vi "TSCAN_SetSignalValue_CANFD.vi"(6 "SigValue":dbl, 7 "TLIBCANFD":T1, 8 "错误输入（无错误）":errorcluster, 9 "Signal":string, 10 "CANFD Message":string, 11 "路径输入":path) -> (0 "错误输出":errorcluster, 1 "CANFDObJ":T1, 2 "return":i32, 3 "路径输出":path)   [LabVIEW 2014]
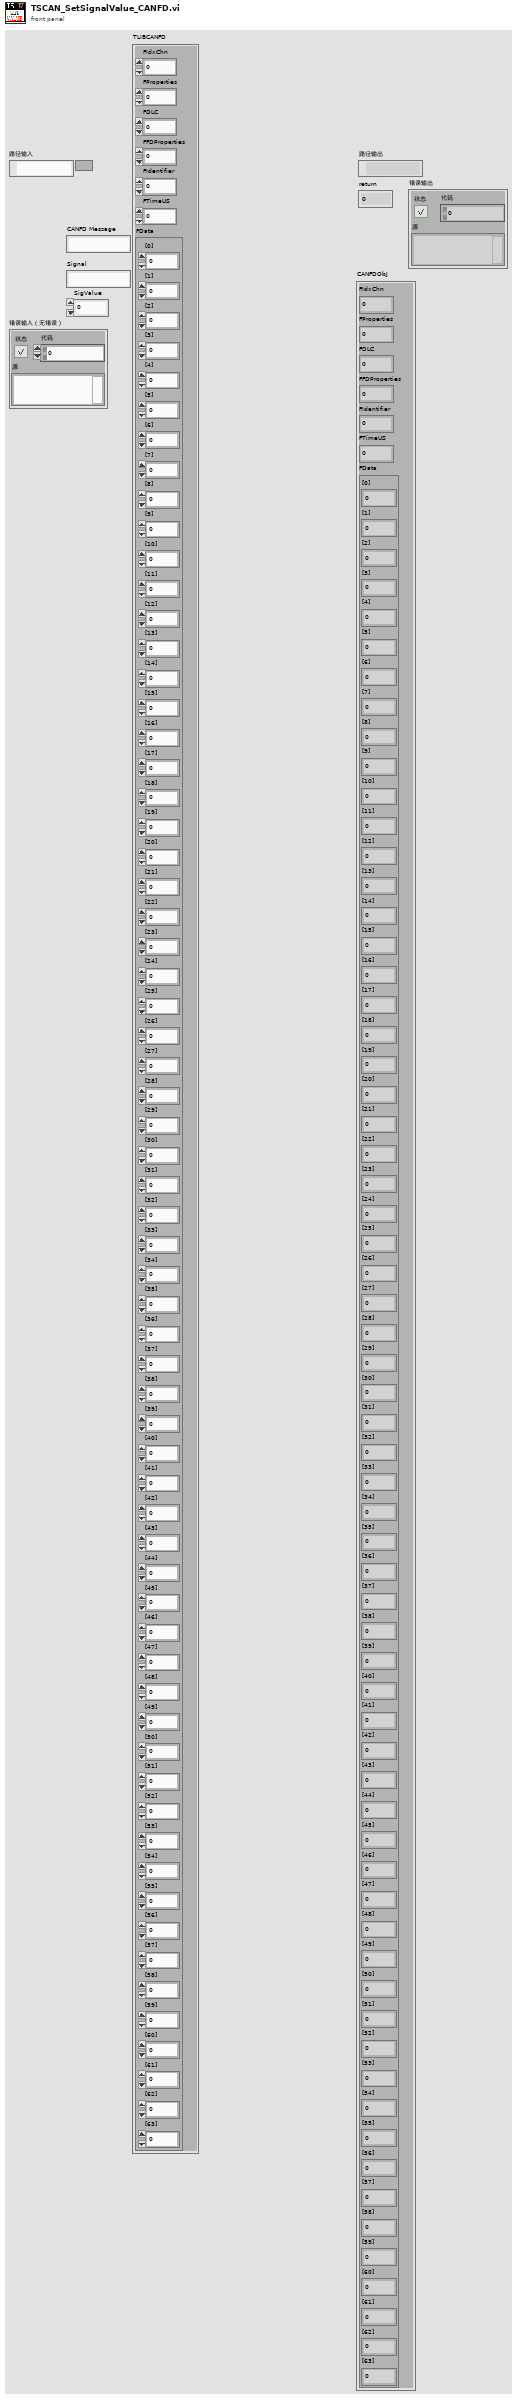
[diagram p1: front panel]
types:
  T1 = cluster{"FIdxChn":u8, "FProperties":u8, "FDLC":u8, "FFDProperties":u8, "FIdentifier":i32, "FTimeUS":u64, "FData":cluster{"[0]":u8, "[1]":u8, "[2]":u8, "[3]":u8, "[4]":u8, "[5]":u8, "[6]":u8, "[7]":u8, "[8]":u8, "[9]":u8, "[10]":u8, "[11]":u8, "[12]":u8, "[13]":u8, "[14]":u8, "[15]":u8, "[16]":u8, "[17]":u8, "[18]":u8, "[19]":u8, "[20]":u8, "[21]":u8, "[22]":u8, "[23]":u8, "[24]":u8, "[25]":u8, "[26]":u8, "[27]":u8, "[28]":u8, "[29]":u8, "[30]":u8, "[31]":u8, "[32]":u8, "[33]":u8, "[34]":u8, "[35]":u8, "[36]":u8, "[37]":u8, "[38]":u8, "[39]":u8, "[40]":u8, "[41]":u8, "[42]":u8, "[43]":u8, "[44]":u8, "[45]":u8, "[46]":u8, "[47]":u8, "[48]":u8, "[49]":u8, "[50]":u8, "[51]":u8, "[52]":u8, "[53]":u8, "[54]":u8, "[55]":u8, "[56]":u8, "[57]":u8, "[58]":u8, "[59]":u8, "[60]":u8, "[61]":u8, "[62]":u8, "[63]":u8}}
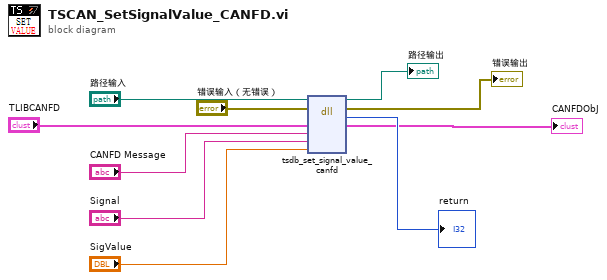
[diagram p0: block diagram]
diagram:
  n1 = dll-call lib="D:/Program Files (x86)/TOSUN/TSMaster/bin/TSMaster.dll" fn="tsdb_set_signal_value_canfd"(path in="路径输入", error in="错误输入（无错误）", "CANObJ"="TLIBCANFD", "Message"="CANFD Message", "Signal"="Signal", "SigValue"="SigValue") -> (path out=→"路径输出":path, error out=→"错误输出":errorcluster, "tsdb_get_signal_value_can"=→"return":i32, "CANObJ"=→"CANFDObJ":T1)  [unwired: 4 in]
